vi "pwmPDT.vi"(8 "error in":errorcluster, 9 "EmergencyStop":refnum<vi>[](array[refnum]), 10 "pwm level / 20":i32, 11 "SetTime / ms":u32) -> (0 "error out":errorcluster)   [LabVIEW 2021]
uses:
  <vilib>/DAQmx/write.llb/DAQmx Write (Analog 1D DBL 1Chan NSamp).vi
  <vilib>/DAQmx/create/channels.llb/DAQmx Create Channel (AO-Voltage-Basic).vi
  <vilib>/DAQmx/configure/timing.llb/DAQmx Timing (Sample Clock).vi
  <vilib>/DAQmx/miscellaneous.llb/DAQmx Fill In Error Info.vi
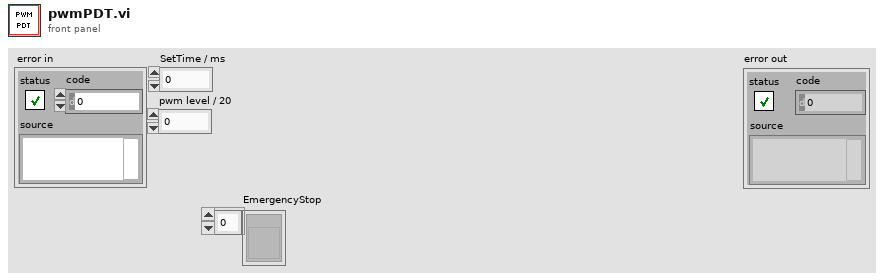
[diagram p1: front panel]
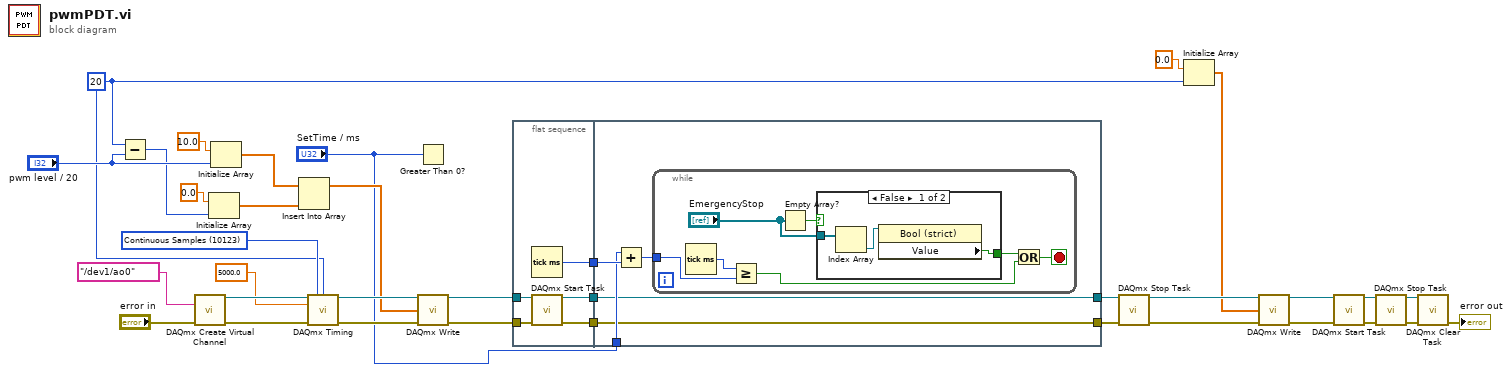
[diagram p0: block diagram]
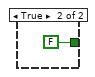
[diagram p2: hidden frame]
diagram:
  w16 = 20 ("samples per channel")
  w27 = 10123 items=["Finite Samples"=10178, "Continuous Samples"=10123, "Hardware Timed Single Point"=12522] ("sample mode")
  n1 = Subtract(x=w16, y="pwm level / 20") -> (x-y=w21:i32)
  n2 = call-poly <vilib>:"DAQmx Create Virtual Channel.vi"("physical channels"=tag "/dev1/ao0", "error in"="error in") -> ("task out"=w32:refnum<k21>, "error out"=w31:errorcluster)  [unwired: 12 in]
  n3 = Initialize Array(0.0 ("element"), w21) -> (w19:dbl[])
  n4 = Initialize Array(10.0 ("element"), "pwm level / 20") -> (w20:dbl[])
  n5 = Insert Into Array(array=w20, new element=w19) -> (w18:dbl[])  [unwired: 1 in]
  n6 = call-poly <vilib>:"DAQmx Timing.vi"("task/channels in"=w32, "sample mode"=w27, "samples per channel"=w16, "rate"=5000.0, "error in"=w31) -> ("task out"=w30:refnum<k21>, "error out"=w29:errorcluster)  [unwired: 9 in]
  n7 = Greater Than 0?(x="SetTime / ms") -> ()  [unwired: 1 out]
  n8 = call-poly <vilib>:"DAQmx Write.vi"("task/channels in"=w30, "data"=w18, "error in"=w29) -> ("task out"=w34:refnum<k21>, "error out"=w33:errorcluster)  [unwired: 10 in, 1 out]
  n9 = flat-sequence {
    tunnel: w34 -> [w40]
    tunnel: w33 -> [w39]
    tunnel: [w38] -> w5
    tunnel: [w37] -> w4
    tunnel: [w36] -> w3
    tunnel: w5 -> [w42]
    tunnel: w4 -> [w41]
    tunnel: w3 -> [w45]
    tunnel: "SetTime / ms" -> [w44]
    tunnel: [w42] -> w2
    tunnel: [w41] -> w1
    frame #0 {
      n10 = Tick Count (ms)() -> (millisecond timer value=w36:u32)
      n11 = call <vilib>:"DAQmx Start Task.vi"("task/channels in"=w40, "error in"=w39) -> ("task out"=w38:refnum<k21>, "error out"=w37:errorcluster)  [unwired: 12 in]
    }
    frame #1 {
      n12 = Add(x=w44, y=w45) -> (x+y=w43:u32)
      n13 = while {
        tunnel: w43 -> [w51]
        stop <- w49 stop-if-true
        n14 = Tick Count (ms)() -> (millisecond timer value=w52:u32)
        n15 = Greater Or Equal?(x=w52, y=w51) -> (x >= y?=w50:bool)
        n16 = Empty Array?(array="EmergencyStop") -> (empty?=w48:bool)
        n17 = case shown="False" w48 {
          tunnel: [w55 FALSE ("Value")] -> w47
          tunnel: "EmergencyStop" -> [w54 _]
          frame False {
            n18 = Index Array(array=w54) -> (element=w53:refnum<vi>)  [unwired: 1 in]
            n19 = property on="Property Node" class="Bool (strict)"(reference=w53) -> ("Value"=w55:bool)  [unwired: 1 in, 2 out]
          }
          frame True {
          }
        }
        n20 = Or(x=w47, y=w50) -> (x .or. y?=w49:bool)
      }
    }
  }
  n21 = call <vilib>:"DAQmx Stop Task.vi"("task/channels in"=w2, "error in"=w1) -> ("task out"=w12:refnum<k21>, "error out"=w13:errorcluster)  [unwired: 12 in]
  n22 = Initialize Array(0.0 ("data"), w16) -> (w9:dbl[])
  n23 = call-poly <vilib>:"DAQmx Write.vi"("task/channels in"=w12, "data"=w9, "error in"=w13) -> ("task out"=w11:refnum<k21>, "error out"=w10:errorcluster)  [unwired: 10 in, 1 out]
  n24 = call <vilib>:"DAQmx Start Task.vi"("task/channels in"=w11, "error in"=w10) -> ("task out"=w14:refnum<k21>, "error out"=w15:errorcluster)  [unwired: 12 in]
  n25 = call <vilib>:"DAQmx Stop Task.vi"("task/channels in"=w14, "error in"=w15) -> ("task out"=w8:refnum<k21>, "error out"=w7:errorcluster)  [unwired: 12 in]
  n26 = call <vilib>:"DAQmx Clear Task.vi"("task in"=w8, "error in"=w7) -> ("error out"=→"error out":errorcluster)  [unwired: 13 in]
